vi "Override To Nominal State.vi"(11 "jettl Actor in":refnum<class "jettl Actor.lvclass">) -> (3 "jettl Actor out":refnum<class "jettl Actor.lvclass">)   [LabVIEW 2021, in "jettl.lvlib" / "Temporary Actor.lvlib" / "jettl Actor.lvclass"]
uses:
  jettl Actor.lvclass
  State.ctl
  jettl Actor.lvclass/jettl Actor.ctl
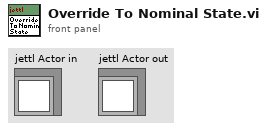
[diagram p1: front panel]
types:
  T1 = typedef "jettl.lvlib/Temporary Actor.lvlib/jettl Actor.lvclass/State.ctl" = enum16{"Nominal", "Teardown", "Error"}
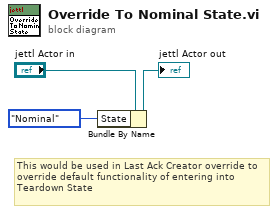
[diagram p0: block diagram]
diagram:
  # "This would be used in Last Ack Creator override to override default functionality of entering into Teardown State"
  n1 = Bundle By Name(cluster="jettl Actor in", "State"=State."Nominal") -> (→"jettl Actor out":refnum<class "jettl Actor.lvclass">)
